vi "Load Audio File.vi"(8 "error in (no error)":errorcluster, 11 "Path":path) -> (0 "error out":errorcluster, 1 "Data":waveform(i16)[](array[waveform]), 2 "Sample Rate (Hz)":u32, 3 "Channels":u32, 5 "Length (Samples)":u64)   [LabVIEW 2019, in "LabVIEW Audio Codecs.lvlib"]
doc: "This VI loads an audio track, placing the audio data into the specified DVR.\n\n<b>Priority:</b> Background\n<b>Execution System:</b> Other 1"
uses:
  LabVIEW Audio Codecs.lvlib
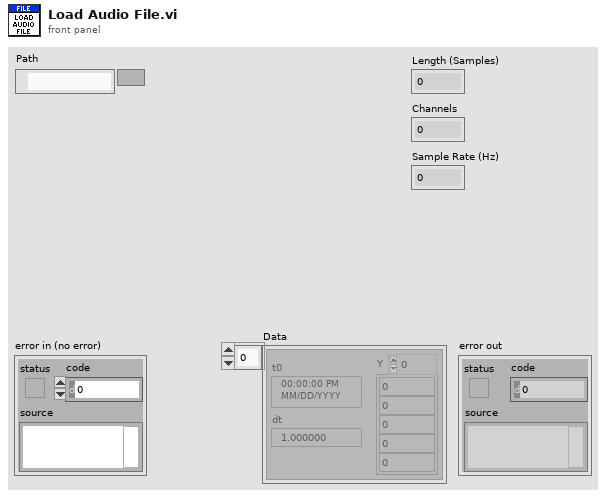
[diagram p1: front panel]
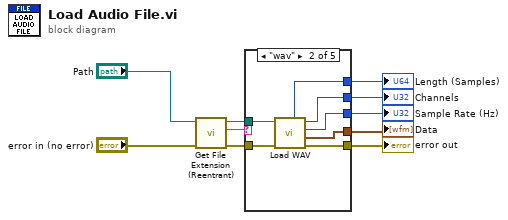
[diagram p0: block diagram]
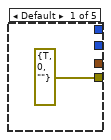
[diagram p2: hidden frame]
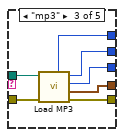
[diagram p3: hidden frame]
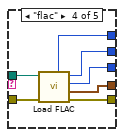
[diagram p4: hidden frame]
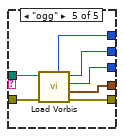
[diagram p5: hidden frame]
diagram:
  n1 = call "Get File Extension (Reentrant).vi"("error in (no error)"="error in (no error)", "file"="Path") -> ("error out"=w8:errorcluster, "lowercase file extension"=w7:string, "dup file"=w6:path)  [unwired: 5 in, 2 out]
  n2 = case shown="\"wav\"" w7 {
    tunnel: w6 -> [_ w17 w25 w32 w39]
    tunnel: w8 -> [_ w18 w24 w31 w38]
    tunnel: [errorcluster {"status"=TRUE, "code"=0, "source"=""} ("error out") w13 w23 w30 w37] -> w5
    tunnel: [_ w14 w22 w29 w36] -> w1
    tunnel: [_ w16 w21 w28 w35] -> w3
    tunnel: [_ w15 w20 w27 w34] -> w2
    tunnel: [_ w12 w19 w26 w33] -> w4
    frame Default {
    }
    frame "wav" {
      n3 = call "Load WAV.vi"("error in (no error)"=w18, "Path"=w17) -> ("error out"=w13:errorcluster, "data"=w14:waveform(i16)[], "Sample Rate (Hz)"=w15:u32, "Channels"=w16:u32, "Length (Samples)"=w12:u64)  [unwired: 5 in]
    }
    frame "mp3" {
      n4 = call "Load MP3.vi"("error in (no error)"=w24, "Path"=w25) -> ("error out"=w23:errorcluster, "data"=w22:waveform(i16)[], "Sample Rate (Hz)"=w20:u32, "Channels"=w21:u32, "Length (Samples)"=w19:u64)  [unwired: 5 in]
    }
    frame "flac" {
      n5 = call "Load FLAC.vi"("error in (no error)"=w31, "Path"=w32) -> ("error out"=w30:errorcluster, "data"=w29:waveform(i16)[], "Sample Rate (Hz)"=w27:u32, "Channels"=w28:u32, "Length (Samples)"=w26:u64)  [unwired: 5 in]
    }
    frame "ogg" {
      n6 = call "Load Vorbis.vi"("error in (no error)"=w38, "Path"=w39) -> ("error out"=w37:errorcluster, "data"=w36:waveform(i16)[], "Sample Rate (Hz)"=w34:u32, "Channels"=w35:u32, "Length (Samples)"=w33:u64)  [unwired: 5 in]
    }
  }
  "error out" <- w5
  "Length (Samples)" <- w4
  "Channels" <- w3
  "Sample Rate (Hz)" <- w2
  "Data" <- w1
